vi "ShowHideControls.vi"(8 "Error In":errorcluster, 9 "Visible":bool, 10 "ControlName":string[](array[string]), 11 "VI Reference":refnum<vi>) -> (0 "Error Out":errorcluster, 3 "VI Reference Out":refnum<vi>)   [LabVIEW 2015]
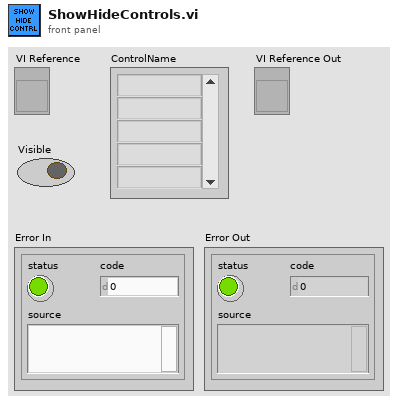
[diagram p1: front panel]
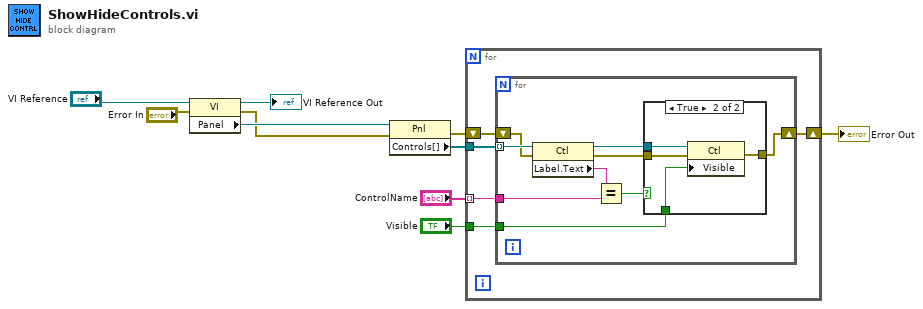
[diagram p0: block diagram]
diagram:
  n1 = property class="VI"(reference="VI Reference", error in="Error In") -> (reference out=→"VI Reference Out":refnum<vi>, error out=w5:errorcluster, "Panel"=w6:refnum<vi>)
  n2 = property class="Pnl"(reference=w6, error in=w5) -> (error out=w3:errorcluster, "Controls[]"=w7:refnum<vi>[])  [unwired: 1 out]
  n3 = for {
    tunnel: w7 -> [w15]
    tunnel: "ControlName" -> [w14] mode=indexing
    tunnel: "Visible" -> [w13]
    shift-right: [w11] -> w2
    shift-left: w3 -> [w12]
    n4 = for {
      tunnel: w15 -> [w24] mode=indexing
      tunnel: w14 -> [w22]
      tunnel: w13 -> [w20]
      shift-right: [w16] -> w11
      shift-left: w12 -> [w18]
      n5 = property class="Ctl"(reference=w24, error in=w18) -> (reference out=w21:refnum<vi>, error out=w17:errorcluster, "Label.Text"=w23:string)
      n6 = Equal?(x=w23, y=w22) -> (x = y?=w19:bool)
      n7 = case shown="True" w19 {
        tunnel: w21 -> [_ w29]
        tunnel: w20 -> [_ w28]
        tunnel: w17 -> [w25 w27]
        tunnel: [w25 w26] -> w16
        frame False {
        }
        frame True {
          n8 = property class="Ctl"(reference=w29, error in=w27, "Visible"=w28) -> (error out=w26:errorcluster)  [unwired: 1 out]
        }
      }
    }
  }
  "Error Out" <- w2
